vi "Choice Dev.vi"(7 "error in":errorcluster caption="错误输入", 10 "Path":string="Config\\data.ini") -> (0 "error out":errorcluster caption="错误输出", 1 "data":string[][](array[string]), 3 "model":string[](array[string]))   [LabVIEW 2013]
uses:
  <vilib>/Utility/config.llb/Read Key (String).vi
  <vilib>/Utility/config.llb/NI_LVConfig.lvlib
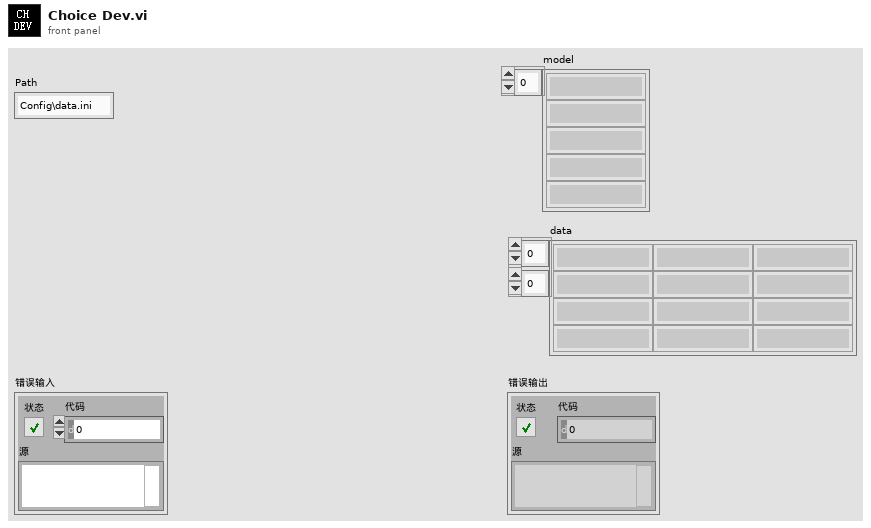
[diagram p1: front panel]
types:
  T1 = enum32{"invalid app kind", "Development System", "Run Time System", "Student Edition", "Embedded LabVIEW", "Evaluation", "Custom"}
  T2 = typedef "NI_LVConfig.lvlib/Config Data RefNum.ctl" = refnum<k1>
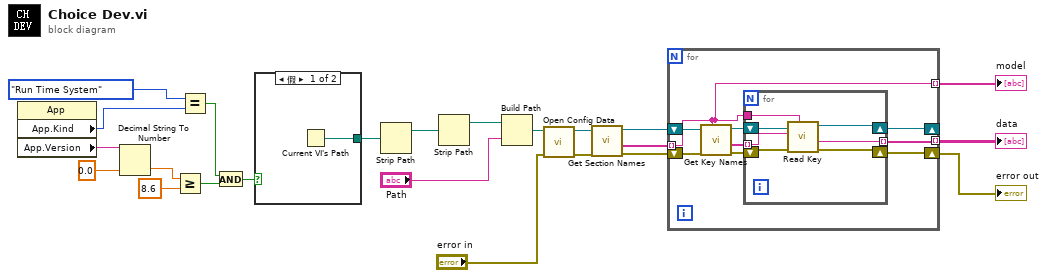
[diagram p0: block diagram]
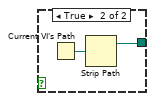
[diagram p2: hidden frame]
diagram:
  n1 = property class="App"() -> ("App.Kind"=w19:T1, "App.Version"=w20:string)  [unwired: 2 in, 2 out]
  n2 = Decimal String To Number(string=w20, default (0L)=0.0 ("y")) -> (number=w22:dbl)  [unwired: 1 in, 1 out]
  n3 = Greater Or Equal?(x=w22, y=8.6) -> (x >= y?=w15:bool)
  n4 = Equal?(x=T1."Run Time System", y=w19) -> (x = y?=w16:bool)
  n5 = And(x=w16, y=w15) -> (x .and. y?=w17:bool)
  n6 = case shown="假" w17 {
    tunnel: [w24 w25] -> w12
    frame False {
      n7 = Current VI's Path() -> (path=w24:path)
    }
    frame True {
      n8 = Current VI's Path() -> (path=w26:path)
      n9 = Strip Path(path=w26) -> (stripped path=w25:path)  [unwired: 1 out]
    }
  }
  n10 = Strip Path(path=w12) -> (stripped path=w11:path)  [unwired: 1 out]
  n11 = Strip Path(path=w11) -> (stripped path=w14:path)  [unwired: 1 out]
  n12 = Build Path(base path=w14, name or relative path="Path") -> (appended path=w10:path)
  n13 = call <vilib>:"Open Config Data.vi"("error in (no error)"="error in", "configuration file path"=w10) -> ("error out"=w8:errorcluster, "refnum"=w9:T2)  [unwired: 7 in, 1 out]
  n14 = call <vilib>:"Get Section Names.vi"("error in (no error)"=w8, "refnum"=w9) -> ("error out"=w6:errorcluster, "section names"=w5:string[], "refnum out"=w7:T2)  [unwired: 7 in]
  n15 = for {
    tunnel: w5 -> [w27] mode=indexing
    shift-right: [w30] -> _
    shift-left: w7 -> [w34]
    shift-right: [w29] -> w1
    shift-left: w6 -> [w35]
    tunnel: [w28] -> w4 mode=indexing
    tunnel: [w27] -> w3 mode=indexing
    n16 = call <vilib>:"Get Key Names.vi"("section"=w27, "error in (no error)"=w35, "refnum"=w34) -> ("error out"=w31:errorcluster, "key names"=w33:string[], "refnum out"=w32:T2)  [unwired: 5 in, 1 out]
    n17 = for {
      tunnel: w33 -> [w41] mode=indexing
      tunnel: w27 -> [w40]
      shift-right: [w37] -> w30
      shift-left: w32 -> [w42]
      shift-right: [w38] -> w29
      shift-left: w31 -> [w39]
      tunnel: [w36] -> w28 mode=indexing
      n18 = call-poly <vilib>:"Read Key.vi"("section"=w40, "error in (no error)"=w39, "key"=w41, "refnum"=w42) -> ("error out"=w38:errorcluster, "value"=w36:string, "refnum out"=w37:T2)  [unwired: 4 in, 1 out]
    }
  }
  "data" <- w4
  "model" <- w3
  "error out" <- w1
